vi "Replace whitespaces.vi"(11 "Text":string) -> (3 "text with spaces replaced":string)   [LabVIEW 2019, in "Panther Dashboard.lvlib"]
uses:
  Panther Dashboard.lvlib
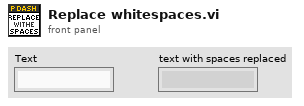
[diagram p1: front panel]
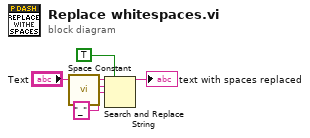
[diagram p0: block diagram]
diagram:
  n1 = call <vilib>:"Space Constant.vi"() -> ("String"=w1:string)
  n2 = Search and Replace String(replace all?=TRUE ("replace all? (F)"), input string="Text", search string=w1, replace string="_") -> (result string=→"text with spaces replaced":string)  [unwired: 4 in, 3 out]
